vi "11111.vi"() -> ()   [LabVIEW 2016]
uses:
  <vilib>/NXT/Subs/LVHSConnector.ctl
  <vilib>/NXT/LegoClasses/BrickReference/BrickReference.lvclass
  <vilib>/NXT/Block Support/NXT_OutputPort.ctl
  <vilib>/NXT/NXTIO Xnodes/NXTIONodeSubVIs/NXTMotorSteeringOn.vi
  <vilib>/NXT/NXTIO Xnodes/AddressXNode/NXTIOAddress.xnode
  <vilib>/NXT/NXTIO Xnodes/NXTIOXNode/NXTIO.xnode
panel:
  in  "NXT/EV3":T1
  in  "Min. speed":i32
  in  "Max. speed":i32
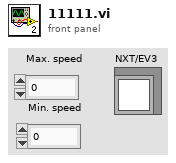
[diagram p1: front panel]
types:
  T1 = typedef "LVHSConnector.ctl" = refnum<class "BrickReference.lvclass">
  T2 = typedef "NXT_OutputPort.ctl" = u8
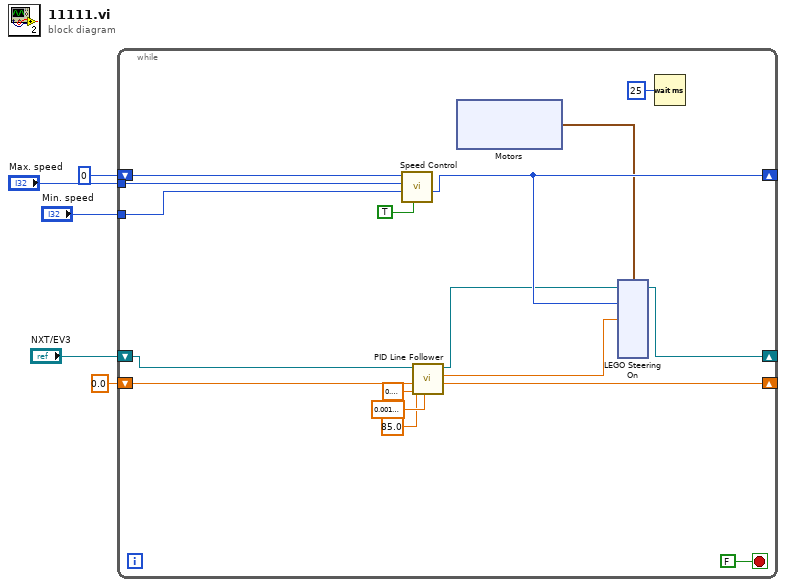
[diagram p0: block diagram]
diagram:
  n1 = while {
    shift-right: [w15] -> _
    shift-left: 0 -> [w22]
    tunnel: "Max. speed" -> [w20]
    tunnel: "Min. speed" -> [w19]
    shift-right: [w16] -> _
    shift-left: sgl 0.0 ("New integral") -> [w17]
    shift-right: [w9] -> _
    shift-left: "NXT/EV3" -> [w10]
    stop <- FALSE stop-if-true
    n2 = call "Speed Control.vi"("Speed Up or Down?"=TRUE, "Min. speed"=w19, "Max. speed"=w20, "Ini. speed"=w22) -> ("Speed out"=w15:i32)  [unwired: 7 in]
    n3 = call "PID Line Follower.vi"("K_i"=sgl 0.001, "K_p"=sgl 0.3, "Previous integral\nerror"=w17, "Target reflection"=sgl 85.0, "EV3 in"=w10) -> ("New integral"=w16:sgl, "Total error"=w12:sgl, "EV3 out"=w13:T1)  [unwired: 4 in]
    n4 = xnode "Motors"() -> ("Motor"=w14:cluster{"Port":T2, "Port":T2})
    n5 = xnode "LEGO Steering On"("Steering 1"=w12, "Power 1"=w15, "Motors"=w14, "NXT/EV3"=w13) -> ("NXT/EV3"=w9:T1)
    n6 = Wait (ms)(milliseconds to wait=u32 25) -> ()  [unwired: 1 out]
  }
